vi "Get Active Worksheet Name.vi"(0 "Report Ref In":T1, 1 "error in (no error)":errorcluster) -> (2 "Report Ref Out":T1, 3 "Worksheet Name":string, 4 "error out":errorcluster)   [LabVIEW 2026, in "XCel Report Engine.lvlib"]
uses:
  XCel Report Engine.lvlib
  Controls/Report Ref.ctl
  C:/Users/m.santucci/Documents/ChatGPT/LV_REPORT_ENGINE/LV/DotNet/XCelReportEngine.dll
  DotNet/XCelReportEngine.dll
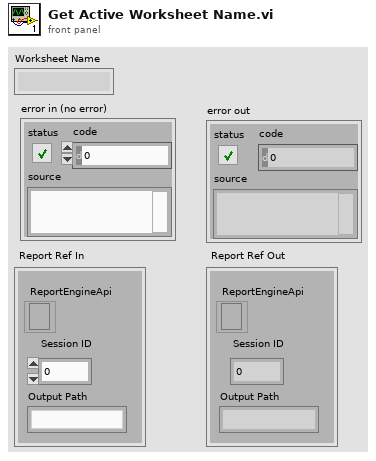
[diagram p1: front panel]
types:
  T1 = typedef "XCel Report Engine.lvlib/Report Ref.ctl" = cluster{"Session ID":i32, "Output Path":string, "ReportEngineApi":refnum<k24>}
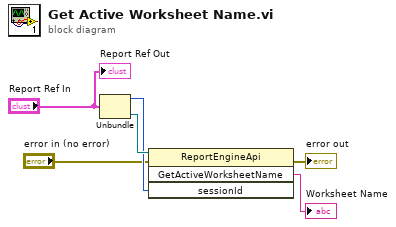
[diagram p0: block diagram]
diagram:
  n1 = Unbundle("Report Ref In") -> ("Session ID"=w4:i32, "ReportEngineApi"=w5:refnum<k24>)  [unwired: 1 out]
  n2 = invoke class="ReportEngineApi" method="GetActiveWorksheetName"(reference=w5, error in="error in (no error)", "sessionId"=w4) -> (error out=→"error out":errorcluster, "GetActiveWorksheetName"=→"Worksheet Name":string)  [unwired: 1 in, 2 out]
  "Report Ref Out" <- "Report Ref In"
